vi "Read Output Definitions and Controller Options.vi"(7 "Unit ID (A)":string="A", 8 "error in":errorcluster, 10 "Software Version":u8, 11 "VISA Session In":refnum<visa-resource-name>="Alicat") -> (0 "error out":errorcluster, 1 "Read-Only Options":T2, 2 "Read/Write Options":T1 {"Controller Select" items=["No controller"=0, "Volumetric Flow"=36, "Mass Flow"=37, "Absolute Pressure"=34, "Gauge Pressure"=38, "Differential Pressure"=39]}, 3 "VISA Session Out":refnum<visa-resource-name>)   [LabVIEW 2024]
doc: "Returns the controller options from the internal configuration registers of an Alicat: selected controller variable, setpoint source, auto tare status, analog setpoint input requirement, variables and voltages of the analog outputs, and whether the control logic is set up for normal or inverse control (labeled pressure or vacuum, respectively due to their common applications)."
panel:
  # "SW Version defaults to 0. \nIf un-wired, it will call a \nsub-VI to check."
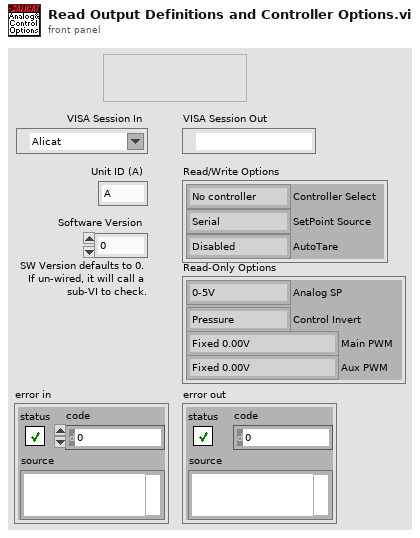
[diagram p1: front panel]
types:
  T1 = cluster{"Controller Select":u16, "SetPoint Source":enum8{"Serial", "Local", "Analog", "Unknown"}, "AutoTare":enum16{"Disabled", "Enabled"}}
  T2 = cluster{"Analog SP":enum16{"0-5V", "4-20mA"}, "Control Invert":enum16{"Pressure", "Vacuum/BP"}, "Main PWM":enum8{"Fixed 0.00V", "Pressure 0-5V", "Temperature 0-5V", "Volumetric Flow 0-5V", "Mass Flow 0-5V", "Pressure 0-2.5-5V bidir", "Temperature 0-2.5-5V bidir", "Volumetric Flow 0-2.5-5V bidir", "Mass Flow 0-2.5-5V bidir", "Pressure 1-5V", "Temperature 1-5V", "Volumetric Flow 1-5V", "Mass Flow 1-5V", "Reserved(A)", "Reserved(B)", "Fixed 5.12V"}, "Aux PWM":enum8{"Fixed 0.00V", "Pressure 0-5V", "Temperature 0-5V", "Volumetric Flow 0-5V", "Mass Flow 0-5V", "Pressure 0-2.5-5V bidir", "Temperature 0-2.5-5V bidir", "Volumetric Flow 0-2.5-5V bidir", "Mass Flow 0-2.5-5V bidir", "Pressure 1-5V", "Temperature 1-5V", "Volumetric Flow 1-5V", "Mass Flow 1-5V", "Reserved(A)", "Reserved(B)", "Fixed 5.12V"}}
  T3 = cluster{"Controller Select":enum8{"No controller", "Pressure", "Temperature", "Volumetric Flow", "Mass Flow", "Unknown"}, "SetPoint Source":enum8{"Serial", "Local", "Analog", "Unknown"}, "AutoTare":enum16{"Disabled", "Enabled"}}
  T4 = enum8{"Fixed 0.00V", "Pressure 0-5V", "Temperature 0-5V", "Volumetric Flow 0-5V", "Mass Flow 0-5V", "Pressure 0-2.5-5V bidir", "Temperature 0-2.5-5V bidir", "Volumetric Flow 0-2.5-5V bidir", "Mass Flow 0-2.5-5V bidir", "Pressure 1-5V", "Temperature 1-5V", "Volumetric Flow 1-5V", "Mass Flow 1-5V", "Reserved(A)", "Reserved(B)", "Fixed 5.12V"}
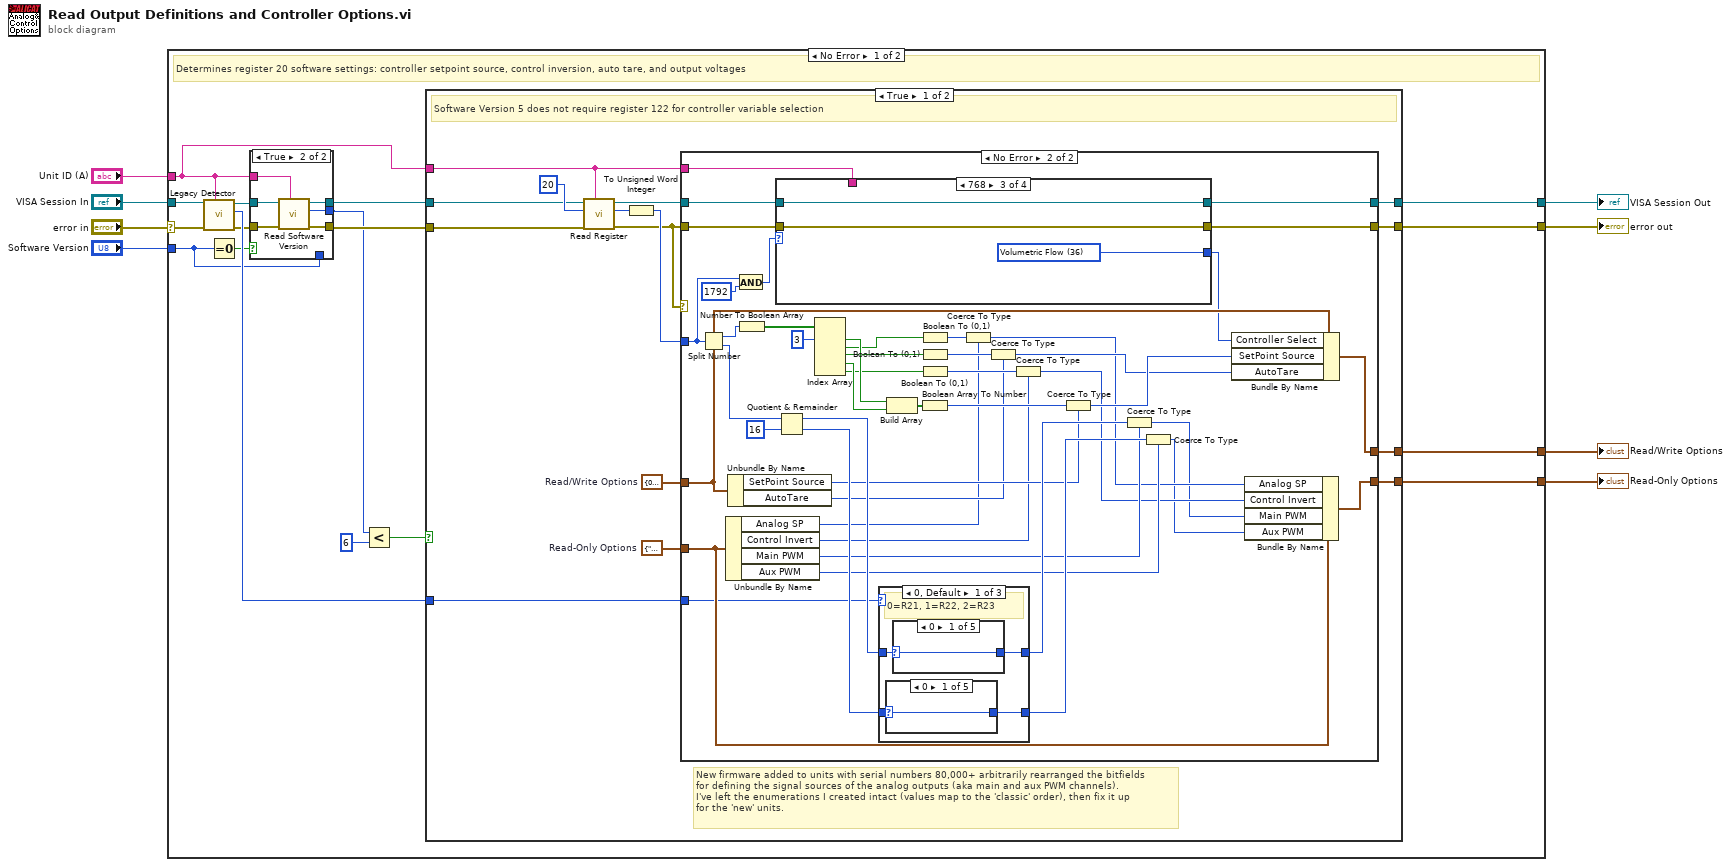
[diagram p0: block diagram]
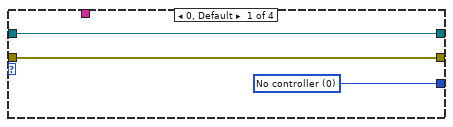
[diagram p4: hidden frame]
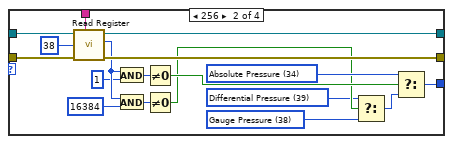
[diagram p5: hidden frame]
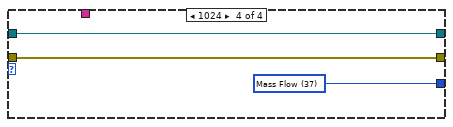
[diagram p6: hidden frame]
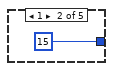
[diagram p7: hidden frame]
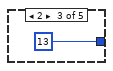
[diagram p8: hidden frame]
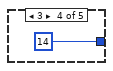
[diagram p9: hidden frame]
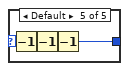
[diagram p10: hidden frame]
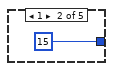
[diagram p11: hidden frame]
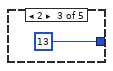
[diagram p12: hidden frame]
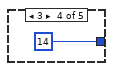
[diagram p13: hidden frame]
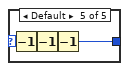
[diagram p14: hidden frame]
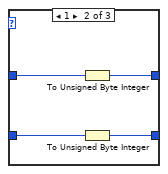
[diagram p15: hidden frame]
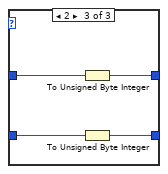
[diagram p16: hidden frame]
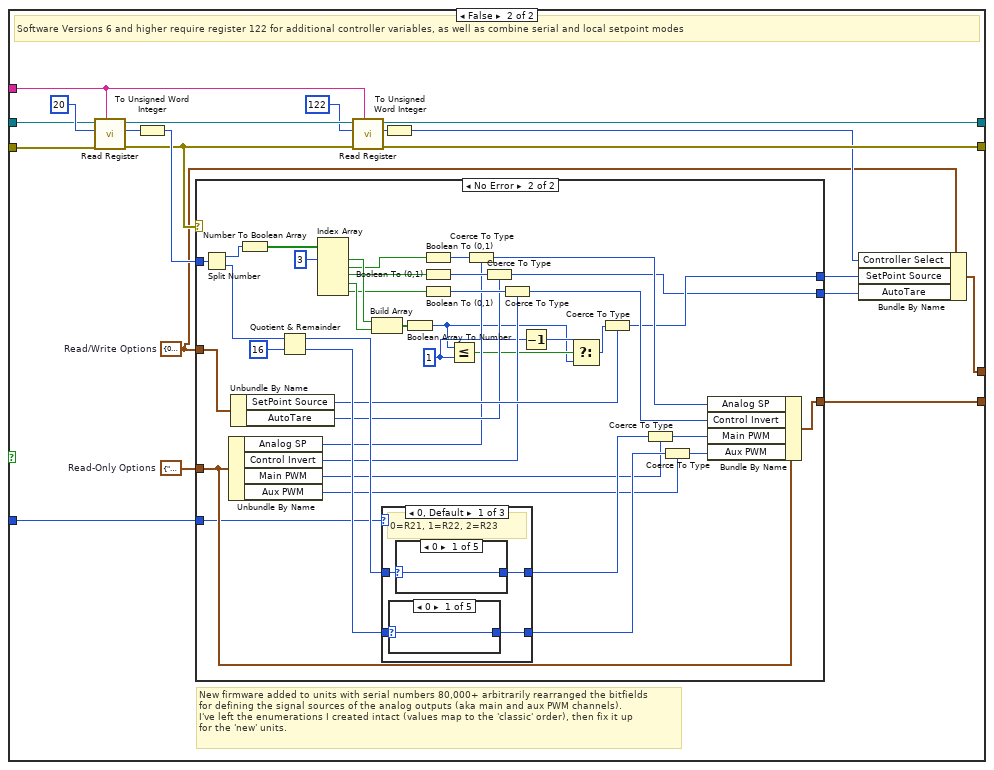
[diagram p17: hidden frame]
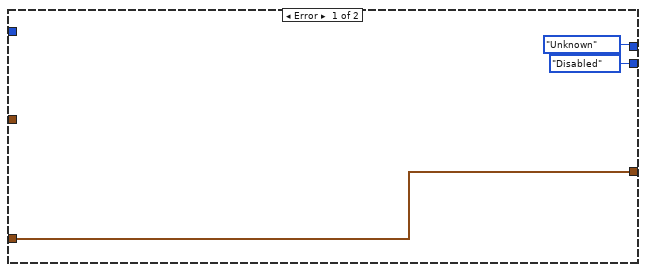
[diagram p18: hidden frame]
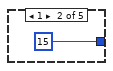
[diagram p19: hidden frame]
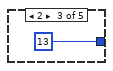
[diagram p20: hidden frame]
diagram:
  n1 = case shown="No Error" "error in" {
    selector: "error in" -> [w19 w247]
    tunnel: [w25 w248] -> w8
    tunnel: [w24 w247] -> w7
    tunnel: [w23 T3 {"Controller Select"=enum."No controller", "SetPoint Source"=enum."Serial", "AutoTare"=enum."Disabled"} ("Read/Write Options")] -> w3
    tunnel: [w22 T2 {"Analog SP"=enum."0-5V", "Control Invert"=enum."Pressure", "Main PWM"=enum."Fixed 0.00V", "Aux PWM"=enum."Fixed 0.00V"} ("Read-Only Options")] -> w2
    tunnel: "VISA Session In" -> [w21 w248]
    tunnel: "Unit ID (A)" -> [w12 _]
    tunnel: "Software Version" -> [w9 _]
    frame No Error {
      # "Determines register 20 software settings: controller setpoint source, control inversion, auto tare, and output voltages"
      n2 = call "Legacy Detector.vi"("Unit ID (A)"=w12, "error in"=w19, "VISA Session In"=w21) -> ("error out"=w16:errorcluster, "Legacy Status"=w20:u8, "VISA Session Out"=w15:refnum<visa-resource-name>)  [unwired: 6 in]
      n3 = Equal To 0?(x=w9) -> (x = 0?=w10:bool)
      n4 = case shown="True" w10 {
        tunnel: w16 -> [w27 w34]
        tunnel: w15 -> [w26 w33]
        tunnel: w12 -> [_ w32]
        tunnel: [w27 w31] -> w13
        tunnel: [w26 w30] -> w14
        tunnel: [w28 w29] -> w11
        tunnel: w9 -> [w28 _]
        frame False {
        }
        frame True {
          n5 = call "Read Software Version.vi"("Unit ID (A)"=w32, "error in"=w34, "VISA Session In"=w33) -> ("error out"=w31:errorcluster, "Software Version"=w29:u8, "VISA Session Out"=w30:refnum<visa-resource-name>)  [unwired: 6 in]
        }
      }
      n6 = Less?(x=w11, y=u8 6) -> (x < y?=w17:bool)
      n7 = case shown="True" w17 {
        tunnel: [w36 w162] -> w25
        tunnel: [w35 w161] -> w24
        tunnel: [w48 w154] -> w23
        tunnel: [w47 w172] -> w22
        tunnel: w20 -> [w46 w171]
        tunnel: w13 -> [w43 w168]
        tunnel: w14 -> [w42 w167]
        tunnel: w12 -> [w38 w163]
        frame True {
          w37 = T1 {"Controller Select"=0, "SetPoint Source"=enum."Serial", "AutoTare"=enum."Disabled"}  # Read/Write Options
          w41 = T2 {"Analog SP"=enum."0-5V", "Control Invert"=enum."Pressure", "Main PWM"=enum."Fixed 0.00V", "Aux PWM"=enum."Fixed 0.00V"}  # Read-Only Options
          # "New firmware added to units with serial numbers 80,000+ arbitrarily rearranged the bitfields\nfor defining the signal sources of the analog outputs (aka main and aux PWM channels).\nI've left the enumerations I created intact (values map to the 'classic' order), then fix it up\nfor the 'new' units."
          # "Software Version 5 does not require register 122 for controller variable selection"
          n8 = call "Read Register.vi"("Unit ID (A)"=w38, "error in"=w43, "Register address"=u16 20 ("register"), "VISA Session In"=w42) -> ("error out"=w39:errorcluster, "Register Value (I32)"=w45:i32, "VISA Session Out"=w40:refnum<visa-resource-name>)  [unwired: 5 in]
          n9 = To Unsigned Word Integer(number=w45) -> (unsigned 16bit integer=w44:u16)
          n10 = case shown="No Error" w39 {
            tunnel: w44 -> [_ w62]
            tunnel: w37 -> [w53 w73]
            tunnel: w46 -> [_ w63]
            tunnel: w41 -> [w52 w72]
            tunnel: [w52 w71] -> w47
            tunnel: [w53 w70] -> w48
            tunnel: w40 -> [w50 w58]
            tunnel: w39 -> [w51 w57]
            tunnel: w38 -> [_ w59]
            tunnel: [w50 w55] -> w36
            tunnel: [w51 w54] -> w35
            frame Error {
            }
            frame No Error {
              n11 = Split Number(x=w62) -> (hi(x)=w97:u8, lo(x)=w95:u8)
              n12 = Unbundle By Name(w72) -> ("Analog SP"=w77:enum16{"0-5V", "4-20mA"}, "Control Invert"=w76:enum16{"Pressure", "Vacuum/BP"}, "Main PWM"=w75:T4, "Aux PWM"=w74:T4)
              n13 = Unbundle By Name(w73) -> ("SetPoint Source"=w79:enum8{"Serial", "Local", "Analog", "Unknown"}, "AutoTare"=w78:enum16{"Disabled", "Enabled"})
              n14 = And(x=w62, y=u16 1792) -> (x .and. y?=w60:u16)
              n15 = Number To Boolean Array(number=w97) -> (Boolean array=w98:bool[])
              n16 = case shown="768" w60 {
                tunnel: w59 -> [_ w119 _ _]
                tunnel: w58 -> [w100 w117 w121 w124]
                tunnel: w57 -> [w101 w118 w122 w125]
                tunnel: [w100 w115 w121 w124] -> w55
                tunnel: [w101 w114 w122 w125] -> w54
                tunnel: [w99 w102 w120 w123] -> w56
                frame 0, Default {
                  w99 = u16 0 items=["No controller"=0, "Volumetric Flow"=36, "Mass Flow"=37, "Absolute Pressure"=34, "Gauge Pressure"=38, "Differential Pressure"=39] ("Controller Select")
                }
                frame 256 {
                  w103 = u16 38 items=["No controller"=0, "Volumetric Flow"=36, "Mass Flow"=37, "Absolute Pressure"=34, "Gauge Pressure"=38, "Differential Pressure"=39] ("Controller Select")
                  w104 = u16 39 items=["No controller"=0, "Volumetric Flow"=36, "Mass Flow"=37, "Absolute Pressure"=34, "Gauge Pressure"=38, "Differential Pressure"=39] ("Controller Select")
                  w109 = u16 34 items=["No controller"=0, "Volumetric Flow"=36, "Mass Flow"=37, "Absolute Pressure"=34, "Gauge Pressure"=38, "Differential Pressure"=39] ("Controller Select")
                  n17 = call "Read Register.vi"("Unit ID (A)"=w119, "error in"=w118, "Register address"=u16 38, "VISA Session In"=w117) -> ("error out"=w114:errorcluster, "Register Value (I32)"=w113:i32, "VISA Session Out"=w115:refnum<visa-resource-name>)  [unwired: 5 in]
                  n18 = And(x=w113, y=1) -> (x .and. y?=w110:i32)
                  n19 = And(x=w113, y=16384) -> (x .and. y?=w107:i32)
                  n20 = Not Equal To 0?(x=w110) -> (x != 0?=w108:bool)
                  n21 = Not Equal To 0?(x=w107) -> (x != 0?=w105:bool)
                  n22 = Select(t=w104, s=w105, f=w103) -> (s? t:f=w106:u16)
                  n23 = Select(t=w109, s=w108, f=w106) -> (s? t:f=w102:u16)
                }
                frame 768 {
                  w120 = u16 36 items=["No controller"=0, "Volumetric Flow"=36, "Mass Flow"=37, "Absolute Pressure"=34, "Gauge Pressure"=38, "Differential Pressure"=39] ("Controller Select")
                }
                frame 1024 {
                  w123 = u16 37 items=["No controller"=0, "Volumetric Flow"=36, "Mass Flow"=37, "Absolute Pressure"=34, "Gauge Pressure"=38, "Differential Pressure"=39] ("Controller Select")
                }
              }
              n24 = Quotient & Remainder(x=w95, y=u8 16) -> (x-y*floor(x/y)=w83:u8, floor(x/y)=w82:u8)
              n25 = Index Array(array=w98, index #1=3 ("idx")) -> (element #1=w92:bool, element #2=w89:bool, element #3=w86:bool, element #4=w91:bool, element #5=w84:bool)  [unwired: 4 in]
              n26 = case shown="0, Default" w63 {
                tunnel: w83 -> [w129 w146 w150]
                tunnel: [w126 w149 w153] -> w80
                tunnel: [w127 w148 w152] -> w81
                tunnel: w82 -> [w128 w147 w151]
                frame 0, Default {
                  # "0=R21, 1=R22, 2=R23"
                  n27 = case shown="0" w128 {
                    selector: w128 -> [w130 _ _ _ w137]
                    tunnel: [w130 u8 15 ("number") u8 13 ("number") u8 14 ("number") w134] -> w127
                    frame 0 {
                    }
                    frame 1 {
                    }
                    frame 2 {
                    }
                    frame 3 {
                    }
                    frame Default {
                      n28 = Decrement(x=w137) -> (x-1=w136:u8)
                      n29 = Decrement(x=w136) -> (x-1=w135:u8)
                      n30 = Decrement(x=w135) -> (x-1=w134:u8)
                    }
                  }
                  n31 = case shown="0" w129 {
                    selector: w129 -> [w138 _ _ _ w145]
                    tunnel: [w138 u8 15 ("number") u8 13 ("number") u8 14 ("number") w142] -> w126
                    frame 0 {
                    }
                    frame 1 {
                    }
                    frame 2 {
                    }
                    frame 3 {
                    }
                    frame Default {
                      n32 = Decrement(x=w145) -> (x-1=w144:u8)
                      n33 = Decrement(x=w144) -> (x-1=w143:u8)
                      n34 = Decrement(x=w143) -> (x-1=w142:u8)
                    }
                  }
                }
                frame 1 {
                  n35 = To Unsigned Byte Integer(number=w146) -> (unsigned 8bit integer=w149:u8)
                  n36 = To Unsigned Byte Integer(number=w147) -> (unsigned 8bit integer=w148:u8)
                }
                frame 2 {
                  n37 = To Unsigned Byte Integer(number=w150) -> (unsigned 8bit integer=w153:u8)
                  n38 = To Unsigned Byte Integer(number=w151) -> (unsigned 8bit integer=w152:u8)
                }
              }
              n39 = Build Array(w92, w91) -> (w93:bool[])
              n40 = Boolean To (0,1)(Boolean=w89) -> (0, 1=w88:i16)
              n41 = Boolean To (0,1)(Boolean=w86) -> (0, 1=w87:i16)
              n42 = Boolean To (0,1)(Boolean=w84) -> (0, 1=w85:i16)
              n43 = Boolean Array To Number(Boolean array=w93) -> (number=w90:u8)
              n44 = Coerce To Type(0:w88, 1:w77) -> (2:w67:enum16{"0-5V", "4-20mA"})
              n45 = Coerce To Type(0:w87, 1:w78) -> (2:w68:enum16{"Disabled", "Enabled"})
              n46 = Coerce To Type(0:w85, 1:w76) -> (2:w66:enum16{"Pressure", "Vacuum/BP"})
              n47 = Coerce To Type(0:w90, 1:w79) -> (2:w69:enum8{"Serial", "Local", "Analog", "Unknown"})
              n48 = Coerce To Type(0:w80, 1:w75) -> (2:w65:T4)
              n49 = Coerce To Type(0:w81, 1:w74) -> (2:w64:T4)
              n50 = Bundle By Name(cluster=w73, "Controller Select"=w56, "SetPoint Source"=w69, "AutoTare"=w68) -> (w70:T1)
              n51 = Bundle By Name(cluster=w72, "Analog SP"=w67, "Control Invert"=w66, "Main PWM"=w65, "Aux PWM"=w64) -> (w71:T2)
            }
          }
        }
        frame False {
          w155 = T1 {"Controller Select"=0, "SetPoint Source"=enum."Unknown", "AutoTare"=enum."Disabled"}  # Read/Write Options
          w166 = T2 {"Analog SP"=enum."0-5V", "Control Invert"=enum."Pressure", "Main PWM"=enum."Fixed 0.00V", "Aux PWM"=enum."Fixed 0.00V"}  # Read-Only Options
          # "New firmware added to units with serial numbers 80,000+ arbitrarily rearranged the bitfields\nfor defining the signal sources of the analog outputs (aka main and aux PWM channels).\nI've left the enumerations I created intact (values map to the 'classic' order), then fix it up\nfor the 'new' units."
          # "Software Versions 6 and higher require register 122 for additional controller variables, as well as combine serial and local setpoint modes"
          n52 = call "Read Register.vi"("Unit ID (A)"=w163, "error in"=w168, "Register address"=u16 20 ("register"), "VISA Session In"=w167) -> ("error out"=w165:errorcluster, "Register Value (I32)"=w170:i32, "VISA Session Out"=w164:refnum<visa-resource-name>)  [unwired: 5 in]
          n53 = To Unsigned Word Integer(number=w170) -> (unsigned 16bit integer=w169:u16)
          n54 = case shown="No Error" w165 {
            tunnel: w169 -> [_ w216]
            tunnel: w171 -> [_ w185]
            tunnel: w166 -> [w176 w191]
            tunnel: [w176 w190] -> w172
            tunnel: w155 -> [_ w179]
            tunnel: [enum8{"Serial", "Local", "Analog", "Unknown"}."Unknown" ("SetPoint Source") w178] -> w157
            tunnel: [enum16{"Disabled", "Enabled"}."Disabled" ("AutoTare") w177] -> w156
            frame Error {
            }
            frame No Error {
              w182 = u8 1 ("y")
              n55 = Split Number(x=w216) -> (hi(x)=w214:u8, lo(x)=w212:u8)
              n56 = Unbundle By Name(w191) -> ("Analog SP"=w195:enum16{"0-5V", "4-20mA"}, "Control Invert"=w194:enum16{"Pressure", "Vacuum/BP"}, "Main PWM"=w193:T4, "Aux PWM"=w192:T4)
              n57 = Unbundle By Name(w179) -> ("SetPoint Source"=w197:enum8{"Serial", "Local", "Analog", "Unknown"}, "AutoTare"=w196:enum16{"Disabled", "Enabled"})
              n58 = Number To Boolean Array(number=w214) -> (Boolean array=w215:bool[])
              n59 = Quotient & Remainder(x=w212, y=u8 16) -> (x-y*floor(x/y)=w201:u8, floor(x/y)=w200:u8)
              n60 = Index Array(array=w215, index #1=3 ("idx")) -> (element #1=w209:bool, element #2=w207:bool, element #3=w204:bool, element #4=w208:bool, element #5=w202:bool)  [unwired: 4 in]
              n61 = Build Array(w209, w208) -> (w210:bool[])
              n62 = case shown="0, Default" w185 {
                tunnel: w201 -> [w220 w237 w241]
                tunnel: [w217 w240 w244] -> w198
                tunnel: [w218 w239 w243] -> w199
                tunnel: w200 -> [w219 w238 w242]
                frame 0, Default {
                  # "0=R21, 1=R22, 2=R23"
                  n63 = case shown="0" w219 {
                    selector: w219 -> [w221 _ _ _ w228]
                    tunnel: [w221 u8 15 ("number") u8 13 ("number") u8 14 ("number") w225] -> w218
                    frame 0 {
                    }
                    frame 1 {
                    }
                    frame 2 {
                    }
                    frame 3 {
                    }
                    frame Default {
                      n64 = Decrement(x=w228) -> (x-1=w227:u8)
                      n65 = Decrement(x=w227) -> (x-1=w226:u8)
                      n66 = Decrement(x=w226) -> (x-1=w225:u8)
                    }
                  }
                  n67 = case shown="0" w220 {
                    selector: w220 -> [w229 _ _ _ w236]
                    tunnel: [w229 u8 15 ("number") u8 13 ("number") u8 14 ("number") w233] -> w217
                    frame 0 {
                    }
                    frame 1 {
                    }
                    frame 2 {
                    }
                    frame 3 {
                    }
                    frame Default {
                      n68 = Decrement(x=w236) -> (x-1=w235:u8)
                      n69 = Decrement(x=w235) -> (x-1=w234:u8)
                      n70 = Decrement(x=w234) -> (x-1=w233:u8)
                    }
                  }
                }
                frame 1 {
                  n71 = To Unsigned Byte Integer(number=w237) -> (unsigned 8bit integer=w240:u8)
                  n72 = To Unsigned Byte Integer(number=w238) -> (unsigned 8bit integer=w239:u8)
                }
                frame 2 {
                  n73 = To Unsigned Byte Integer(number=w241) -> (unsigned 8bit integer=w244:u8)
                  n74 = To Unsigned Byte Integer(number=w242) -> (unsigned 8bit integer=w243:u8)
                }
              }
              n75 = Boolean Array To Number(Boolean array=w210) -> (number=w181:u8)
              n76 = Boolean To (0,1)(Boolean=w207) -> (0, 1=w206:i16)
              n77 = Boolean To (0,1)(Boolean=w204) -> (0, 1=w205:i16)
              n78 = Boolean To (0,1)(Boolean=w202) -> (0, 1=w203:i16)
              n79 = Less Or Equal?(x=w181, y=w182) -> (x <= y?=w184:bool)
              n80 = Coerce To Type(0:w206, 1:w195) -> (2:w189:enum16{"0-5V", "4-20mA"})
              n81 = Coerce To Type(0:w205, 1:w196) -> (2:w177:enum16{"Disabled", "Enabled"})
              n82 = Coerce To Type(0:w203, 1:w194) -> (2:w188:enum16{"Pressure", "Vacuum/BP"})
              n83 = Decrement(x=w182) -> (x-1=w183:u8)
              n84 = Select(t=w183, s=w184, f=w181) -> (s? t:f=w180:u8)
              n85 = Coerce To Type(0:w180, 1:w197) -> (2:w178:enum8{"Serial", "Local", "Analog", "Unknown"})
              n86 = Coerce To Type(0:w198, 1:w193) -> (2:w187:T4)
              n87 = Coerce To Type(0:w199, 1:w192) -> (2:w186:T4)
              n88 = Bundle By Name(cluster=w191, "Analog SP"=w189, "Control Invert"=w188, "Main PWM"=w187, "Aux PWM"=w186) -> (w190:T2)
            }
          }
          n89 = call "Read Register.vi"("Unit ID (A)"=w163, "error in"=w165, "Register address"=u16 122, "VISA Session In"=w164) -> ("error out"=w161:errorcluster, "Register Value (I32)"=w159:i32, "VISA Session Out"=w162:refnum<visa-resource-name>)  [unwired: 5 in]
          n90 = To Unsigned Word Integer(number=w159) -> (unsigned 16bit integer=w158:u16)
          n91 = Bundle By Name(cluster=w155, "Controller Select"=w158, "SetPoint Source"=w157, "AutoTare"=w156) -> (w154:T1)
        }
      }
    }
    frame Error {
    }
  }
  "error out" <- w7
  "VISA Session Out" <- w8
  "Read-Only Options" <- w2
  "Read/Write Options" <- w3
